vi "FourFlippingCoins.vi"() -> ()   [LabVIEW 2014]
uses:
  <vilib>/Analysis/NI_AALBase.lvlib
panel:
  out "Waveform Graph":cluster{i32, i32, "Histogram: h(x)":i32[]}(graph)
  out "Array":i16[](array[numeric])
  in  "Number of Trials":dbl
  out "Number of Heads":dbl
  out "Coin 4":bool
  out "Coin 3":bool
  out "Coin 2":bool
  out "Coin 1":bool
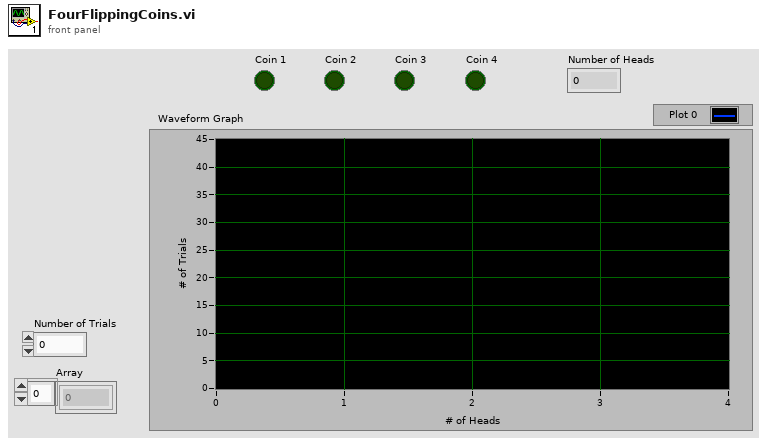
[diagram p1: front panel]
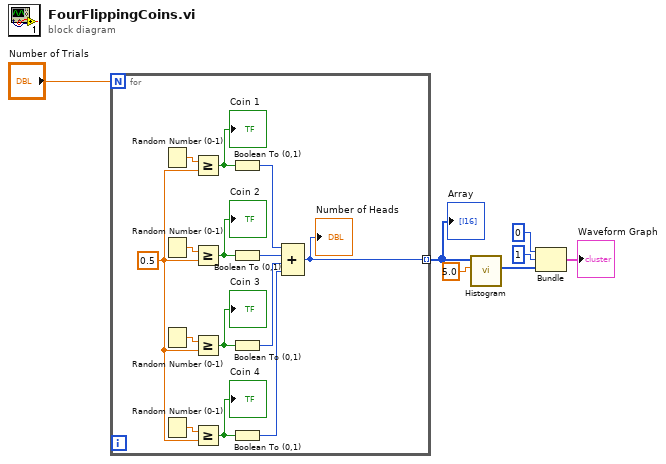
[diagram p0: block diagram]
diagram:
  n1 = for {
    N: "Number of Trials" -> [_]
    tunnel: [w8] -> w6 mode=indexing
    w17 = 0.5
    n2 = Random Number (0-1)() -> (number: 0 to 1=w20:dbl)
    n3 = Random Number (0-1)() -> (number: 0 to 1=w18:dbl)
    n4 = Random Number (0-1)() -> (number: 0 to 1=w15:dbl)
    n5 = Random Number (0-1)() -> (number: 0 to 1=w16:dbl)
    n6 = Greater Or Equal?(x=w20, y=w17) -> (x >= y?=w19:bool)
    "Coin 1" <- w19
    n7 = Greater Or Equal?(x=w18, y=w17) -> (x >= y?=w10:bool)
    "Coin 2" <- w10
    n8 = Greater Or Equal?(x=w15, y=w17) -> (x >= y?=w11:bool)
    "Coin 3" <- w11
    n9 = Greater Or Equal?(x=w16, y=w17) -> (x >= y?=w9:bool)
    "Coin 4" <- w9
    n10 = Boolean To (0,1)(Boolean=w19) -> (0, 1=w21:i16)
    n11 = Boolean To (0,1)(Boolean=w10) -> (0, 1=w12:i16)
    n12 = Boolean To (0,1)(Boolean=w11) -> (0, 1=w13:i16)
    n13 = Boolean To (0,1)(Boolean=w9) -> (0, 1=w14:i16)
    n14 = Compound Arithmetic op=ADD(w21, w12, w13, w14) -> (w8:i16)
    "Number of Heads" <- w8
  }
  "Array" <- w6
  n15 = call <vilib>:"Histogram.vi"("intervals"=5.0, "X"=w6) -> ("Histogram: h(x)"=w1:i32[])  [unwired: 6 in, 3 out]
  n16 = Bundle(0, 1, "Histogram: h(x)"=w1) -> (→"Waveform Graph":cluster{i32, i32, "Histogram: h(x)":i32[]})  [unwired: 1 in]
